vi "Double FFT Mesurament RT with TIME Linearization (Not working mehtod).vi"() -> ()   [LabVIEW 2014]
uses:
  <vilib>/Platform/TimedLoop/XDataNode/timing_clust.ctl
  <vilib>/Platform/TimedLoop/XDataNode/nitl_modes.ctl
  <vilib>/Platform/TimedLoop/XDataNode/wakeup.ctl
  <vilib>/FPGAPlugInAG/sbRIO-9636/niLvFpga_Open_sbRIO-9636.vi
  <vilib>/rvi/interface/common/dynamic/niFpgaDynamicAddResources.vi
  <vilib>/Utility/error.llb/Error Cluster From Error Code.vi
  <vilib>/rvi/errors/niLvFpgaAdjustHostInterfaceError.vi
  <vilib>/rvi/interface/common/niFpgaWaitOnOcc.vi
  <vilib>/FPGAPlugInAG/Dynamic/niLvFpga_Run_Dynamic.vi
  <vilib>/FPGAPlugInAG/Dynamic/niLvFpga_Abort_Dynamic.vi
  <vilib>/FPGAPlugInAG/Dynamic/niLvFpga_Reset_Dynamic.vi
  <vilib>/FPGAPlugInAG/Dynamic/niLvFpga_Close_Dynamic.vi
  <vilib>/rvi/interface/nirviOpenFPGA/nirviOpenFPGA.xnode
  FPGA Bitfiles/LaserDistanceSen_FPGATarget_DoubleFFTMesuram_r82pz3ZO4sk.lvbitx
  FPGA Target/Test VIs/Double FFT Mesurament Test.vi
  <vilib>/rvi/interface/nirviReadWriteControl/nirviReadWriteControl.xnode
  <vilib>/rvi/interface/nirviMethod/nirviMethod.xnode
  <vilib>/Platform/TimedLoop/XDataNode/XDataNode.xnode
  <vilib>/rvi/interface/nirviCloseFPGA/nirviCloseFPGA.xnode
  <vilib>/FPGAPlugInAG/Dynamic/niLvFpga_ConfigureFifo_Dynamic.vi
  <vilib>/rvi/errors/niLvFpgaMergeErrorWithErrorCode.vi
  <vilib>/FPGAPlugInAG/Dynamic/niLvFpga_StartFifo_Dynamic.vi
  <vilib>/rvi/interface/Simulation/niFpgaSimulationCallBeginRW.vi
  <vilib>/FPGAPlugInAG/Dynamic/niLvFpga_ReadFifo_Dynamic.vi
  <vilib>/Platform/TimedLoop/XDataNode/XDNodeRunTimeDep.lvlib
  NiFpgaLv.dll
panel:
  in  "tieni premuto per":i32=1
  out "Not-Extended Period Fal":cluster{"yi":dbl[], "yi":dbl[]}(graph)
  out "Not-Extended Period RIs":cluster{"yi":dbl[], "yi":dbl[]}(graph)
  out "Triangular Signal (ris-fal)":dbl[](graph)
  out "current lin":i32
  out "Triangular Signal (fal-ris)":dbl[](graph)
  out "Period Graph Ris":dbl[][](graph)
  out "Period Graph Fall":dbl[][](graph)
  in  "Acrive Linearization":bool
  out "#Peaks Sig2":i32
  out "#Peaks Sig1":i32
  in  "polynomial order":i32=3
  in  "side points":i32=13
  out "Second Signal SMOOTH":dbl[](graph)
  out "First Signal SMOOTH":dbl[](graph)
  in  "# Measurements for Linearization":i32=10
  in  "stop":bool
  out "maxbin_secondFFT":i32
  out "maxbin_firstFFT":i32
  out "f_rise":dbl
  out "f_fall":dbl
  out "f_mean":dbl
  out "Velocity (m/s)":dbl
  out "Distance (m)":dbl
  in  "Initial Latency points":u32(slide)=10 scale=0.0..1249.0
  out "Second FFT (bin)":dbl[](graph)
  out "Second Signal (points) - Rising Triangular":dbl[](graph)
  out "First FFT (bin)":dbl[](graph)
  out "First Signal (points) - Falling Triangular":dbl[](graph)
  in  "Snapshot":bool
  in  "Windowing":T1(ring)
  in  "first bin":i32=5
  in  "last bin":i32=255
  in  "lower limit 2":u32(slide)=725 scale=625.0..738.0
  in  "lower limit 1":u32(slide)=100 scale=0.0..113.0
  # "WARNING:\nOnce pressed wait untill the end of operation"
  # "OFFLINE parameters"
  # "Max Detection FFT bin range"
  # "S-G Parameter for Smoothing"
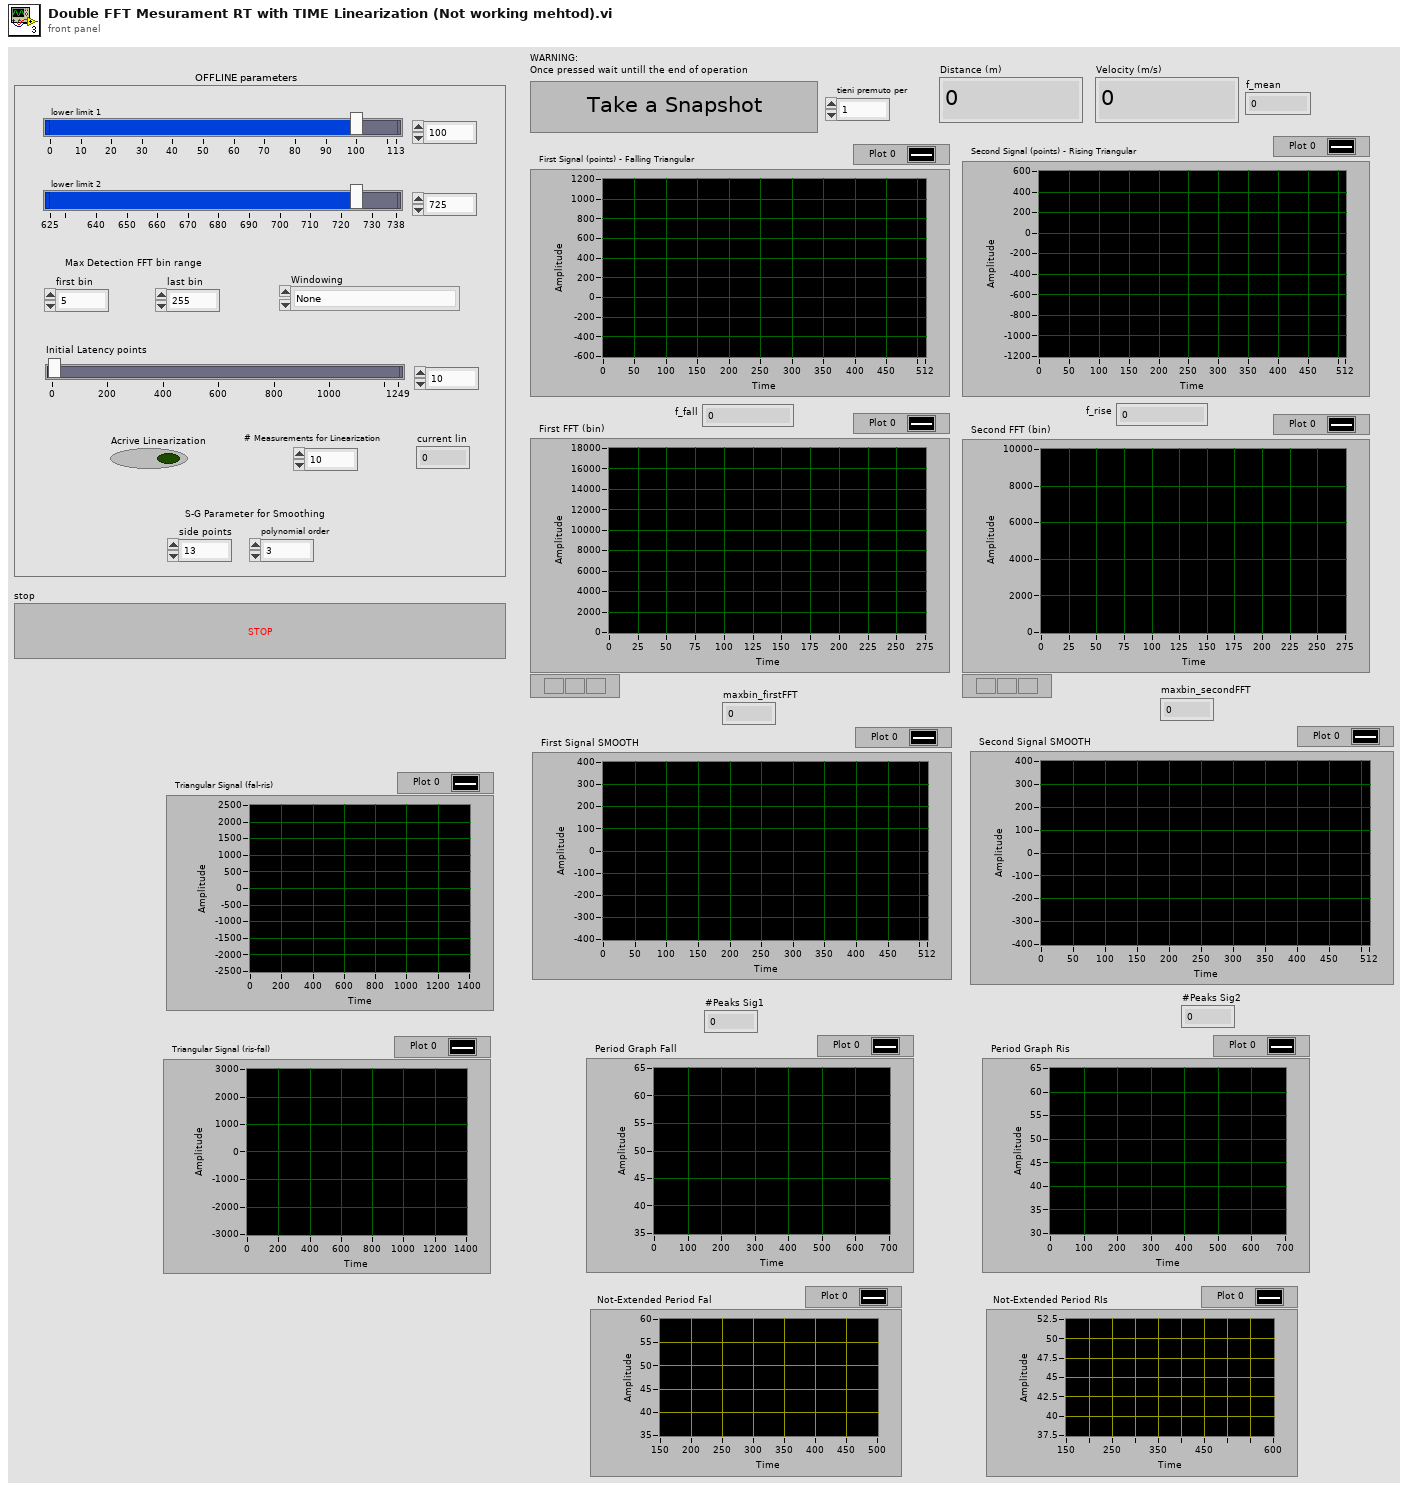
[diagram p1: front panel]
types:
  T1 = enum16{"None", "Hanning", "Hamming", "Blackman", "Blackman-Harris"}
  T2 = typedef "XDNodeRunTimeDep.lvlib/timing_clust.ctl" = cluster{"Expected End [f-1]":u64, "Actual End [f-1]":u64, "Finished Late? [f-1]":bool, "Expected End [i-1]":u64, "Actual End [i-1]":u64, "Finished Late? [i-1]":bool, "Expected Start [i]":u64, "Actual Start [i]":u64, "Expected Start [f]":u64, "Actual Start [f]":u64, "Source Name":string, "Structure Name":string, "Period":i64, "Deadline":i64, "Offset":i64, "Start":i64, "Priority":i32, "Timeout":i32, "Mode":T3, "Wakeup Reason":T4, "Error":errorcluster, "Source Type":string, "Secondary Source Type":string, "Global End Time":u64, "Global Start Time":u64, "Frame Duration":u64, "Iteration Duration":u64, "Assigned CPU":i32, "I/O Scan Engine Mode":u32}
  T3 = typedef "XDNodeRunTimeDep.lvlib/nitl_modes.ctl" = enum32{"No Change", "Process missed periods, maintain original phase", "Discard missed periods, maintain original phase", "Process missed periods, ignore original phase", "Discard missed periods, ignore original phase"}
  T4 = typedef "XDNodeRunTimeDep.lvlib/wakeup.ctl" = enum32{"Normal", "Aborted", "Asynchronous wakeup", "Timing source error", "Timed loop error", "Timeout"}
  T5 = typedef "NI_Matrix.lvlib/RealMatrix.ctl" = dbl[][]
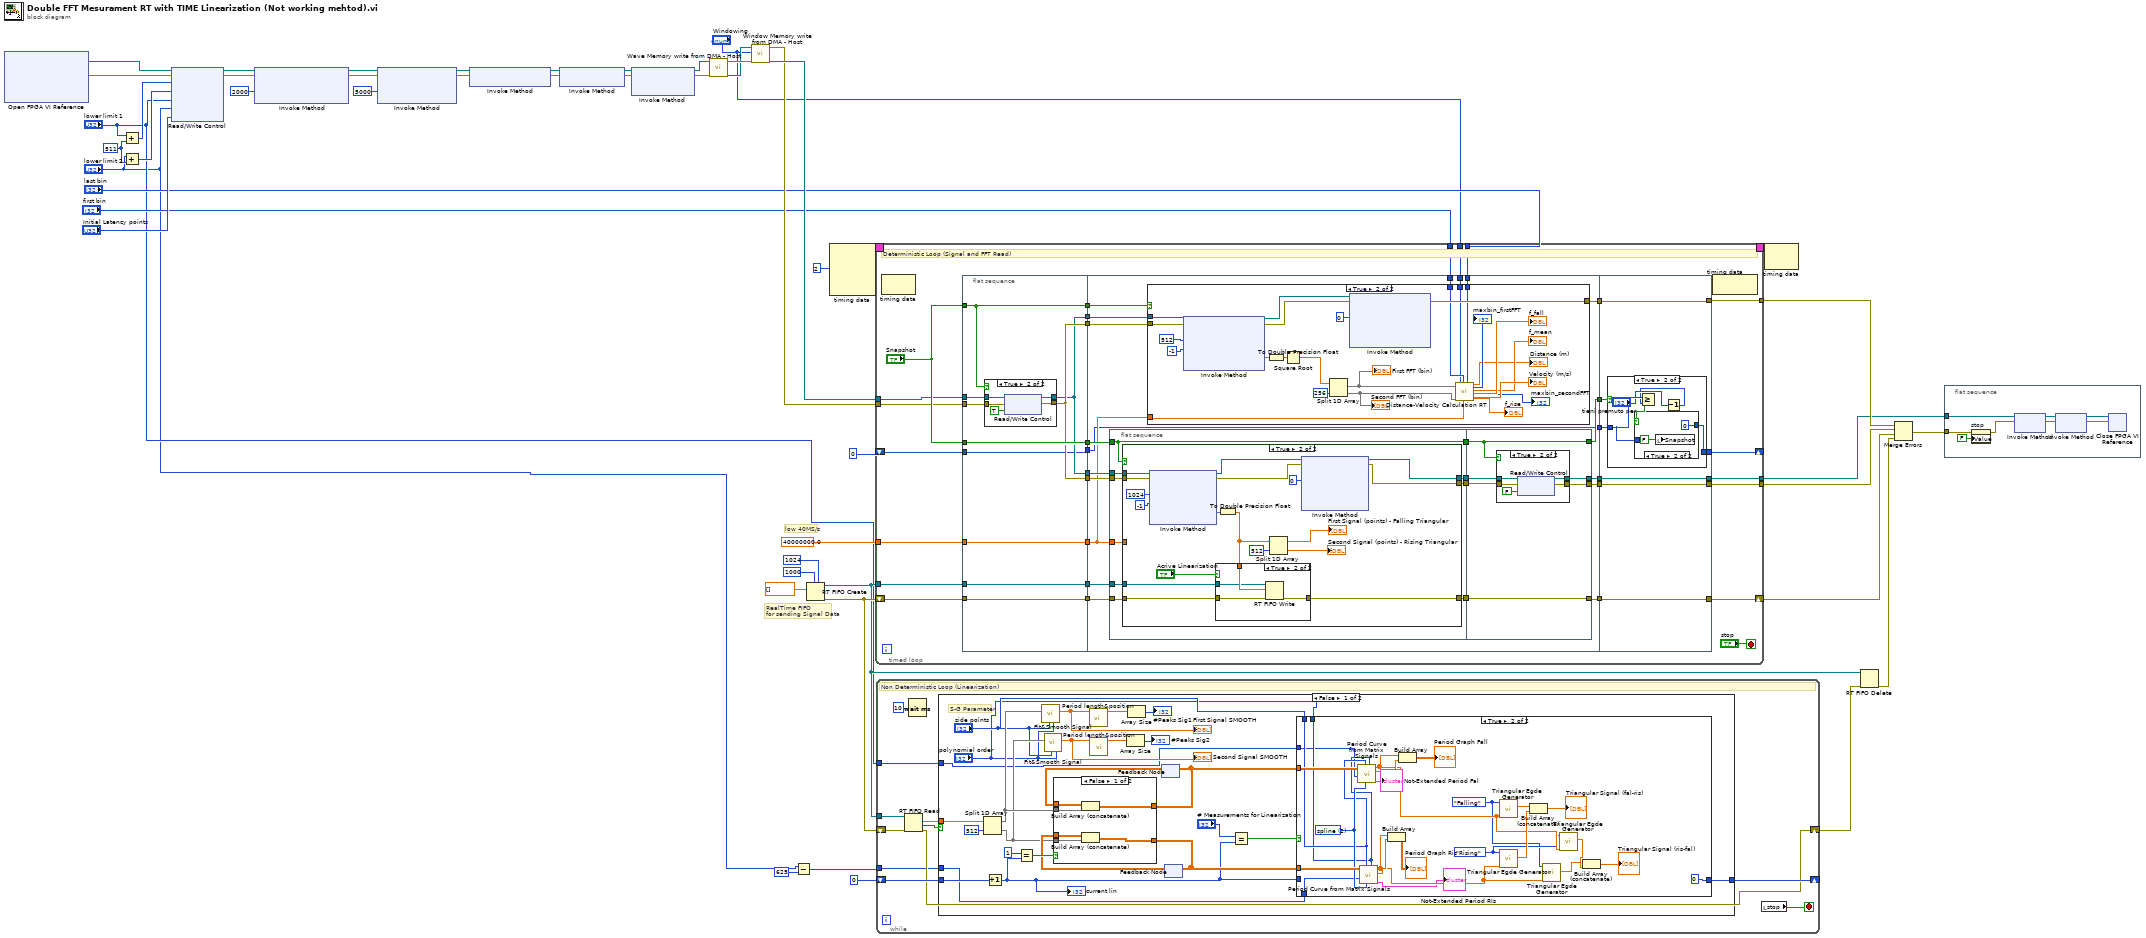
[diagram p0: block diagram]
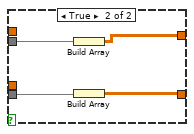
[diagram p3: hidden frame]
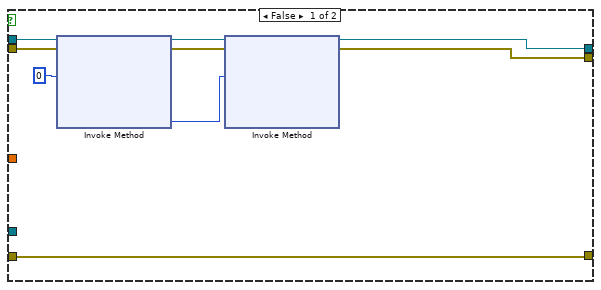
[diagram p6: hidden frame]
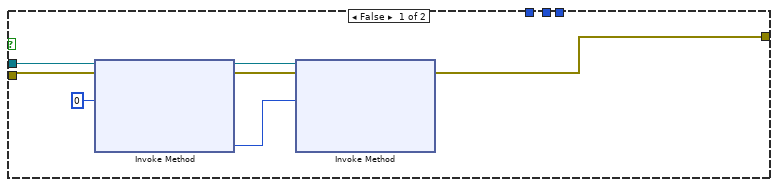
[diagram p9: hidden frame]
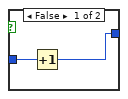
[diagram p11: hidden frame]
diagram:
  w47 = u32 511 ("y")
  # "RealTime FIFO \nfor sending Signal Data"
  # "low 40MS/s"
  n1 = xnode "Open FPGA VI Reference"() -> ("FPGA VI Reference Out"=w46:refnum<k20>, "error out"=w45:errorcluster)  [unwired: 2 in]
  n2 = Add(x="lower limit 1", y=w47) -> (x+y=w49:u32)
  n3 = Add(x="lower limit 2", y=w47) -> (x+y=w48:u32)
  n4 = xnode "Read/Write Control"("FPGA VI Reference In"=w46, "error in"=w45, "upper limit 1"=w49, "upper limit 2"=w48, "lower limit 1"="lower limit 1", "lower limit 2"="lower limit 2", "Latency points"="Initial Latency points") -> ("FPGA VI Reference Out"=w42:refnum<k20>, "error out"=w41:errorcluster)
  n5 = xnode "Invoke Method"("FPGA VI Reference In"=w42, "error in"=w41, "Requested Depth"=u32 2000) -> ("FPGA VI Reference Out"=w20:refnum<k20>, "error out"=w21:errorcluster)  [unwired: 1 out]
  n6 = xnode "Invoke Method"("FPGA VI Reference In"=w20, "error in"=w21, "Requested Depth"=u32 5000) -> ("FPGA VI Reference Out"=w34:refnum<k20>, "error out"=w35:errorcluster)  [unwired: 1 out]
  n7 = xnode "Invoke Method"("FPGA VI Reference In"=w34, "error in"=w35) -> ("FPGA VI Reference Out"=w18:refnum<k20>, "error out"=w19:errorcluster)
  n8 = xnode "Invoke Method"("FPGA VI Reference In"=w18, "error in"=w19) -> ("FPGA VI Reference Out"=w32:refnum<k20>, "error out"=w33:errorcluster)
  n9 = xnode "Invoke Method"("FPGA VI Reference In"=w32, "error in"=w33) -> ("FPGA VI Reference Out"=w38:refnum<k20>, "error out"=w37:errorcluster)  [unwired: 1 in]
  n10 = call "Wave Memory write from DMA - Host.vi"("error in"=w37, "FPGA VI Reference In"=w38) -> ("FPGA VI Reference Out"=w23:refnum<k20>, "error out"=w36:errorcluster)  [unwired: 7 in, 1 out]
  n11 = call "Window Memory write from DMA - Host.vi"("error in"=w36, "Enum"="Windowing", "FPGA VI Reference In"=w23) -> ("FPGA VI Reference Out"=w44:refnum<k20>, "error out"=w43:errorcluster)  [unwired: 5 in, 2 out]
  n12 = Subtract(x="lower limit 2", y=u32 625) -> (x-y=w2:u32)
  n13 = RT FIFO Create(1:dbl[] [] ("double precision float"), 4:u32 1000 ("size (10)"), 6:u32 1024 ("elements in array (1)")) -> (8:w10:refnum<k33>, 11:w12:errorcluster)  [unwired: 5 in, 1 out]
  n14 = node-c288(i64 2 ("Period")) -> (w31:T2)  [unwired: 3 in]
  n15 = timed-loop {
    tunnel: w44 -> [w76]
    tunnel: w43 -> [w77]
    tunnel: [w79] -> w28
    tunnel: 40000000.0 ("Sample Rate (S/s)") -> [w81]
    tunnel: [w80] -> w27
    timing: w31 -> [_]
    timing-out: [_] -> w30
    tunnel: "first bin" -> [w65]
    tunnel: "last bin" -> [w64]
    tunnel: [w62] -> w22
    tunnel: "Windowing" -> [w60]
    shift-right: [w54] -> w13
    shift-left: w12 -> [w56]
    tunnel: w10 -> [w58]
    shift-right: [w50] -> _
    shift-left: 0 -> [w52]
    stop <- "stop" stop-if-true
    # "Deterministic Loop (Signal and FFT Read)"
    n16 = node-c288() -> ()  [unwired: 1 in, 1 out]
    n17 = flat-sequence {
      tunnel: w76 -> [w89]
      tunnel: w77 -> [w90]
      tunnel: "Snapshot" -> [w87]
      tunnel: "Snapshot" -> [w92]
      tunnel: w81 -> [w93]
      tunnel: [w91] -> w75
      tunnel: [w93] -> w74
      tunnel: [w92] -> w73
      tunnel: [w87] -> w72
      tunnel: [w91] -> w71
      tunnel: [w88] -> w70
      tunnel: [w88] -> w69
      tunnel: [w86] -> w59
      tunnel: w58 -> [w86]
      tunnel: [w85] -> w57
      tunnel: w56 -> [w85]
      tunnel: [w84] -> w53
      tunnel: w52 -> [w84]
      tunnel: w75 -> [w118]
      tunnel: w74 -> [w106]
      tunnel: w73 -> [w112]
      tunnel: w72 -> [w115]
      tunnel: w71 -> [w114]
      tunnel: w70 -> [w113]
      tunnel: w69 -> [w119]
      tunnel: [w117] -> w68
      tunnel: [w116] -> w67
      tunnel: [w111] -> w66
      tunnel: w65 -> [w110]
      tunnel: w64 -> [w109]
      tunnel: [w108] -> w61
      tunnel: w60 -> [w107]
      tunnel: w59 -> [w105]
      tunnel: w57 -> [w104]
      tunnel: [w102] -> w55
      tunnel: w53 -> [w101]
      tunnel: [w101] -> w51
      tunnel: [w214] -> w79
      tunnel: [w215] -> w80
      tunnel: w68 -> [w215]
      tunnel: w67 -> [w214]
      tunnel: w66 -> [w213]
      tunnel: [w212] -> w62
      tunnel: w61 -> [w212]
      tunnel: [w211] -> w54
      tunnel: w55 -> [w211]
      tunnel: w51 -> [w210]
      tunnel: [w209] -> w50
      frame #0 {
        n18 = case shown="True" w87 {
          tunnel: [w94 w99] -> w91
          tunnel: w90 -> [w94 w98]
          tunnel: w89 -> [w95 w97]
          tunnel: [w95 w96] -> w88
          frame False {
          }
          frame True {
            n19 = xnode "Read/Write Control"("FPGA VI Reference In"=w97, "error in"=w98, "snapshot"=TRUE) -> ("FPGA VI Reference Out"=w96:refnum<k20>, "error out"=w99:errorcluster)
          }
        }
      }
      frame #1 {
        n20 = flat-sequence {
          tunnel: w119 -> [w131]
          tunnel: w118 -> [w130]
          tunnel: w106 -> [w129]
          tunnel: w112 -> [w126]
          tunnel: [w128] -> w122
          tunnel: [w127] -> w121
          tunnel: [w126] -> w120
          tunnel: w105 -> [w125]
          tunnel: w104 -> [w124]
          tunnel: [w123] -> w103
          tunnel: [w167] -> w116
          tunnel: w122 -> [w169]
          tunnel: w121 -> [w168]
          tunnel: w120 -> [w166]
          tunnel: [w166] -> w111
          tunnel: [w165] -> w108
          tunnel: [w164] -> w102
          tunnel: w103 -> [w164]
          frame #0 {
            n21 = case shown="True" w126 {
              tunnel: w131 -> [w139 w158]
              tunnel: w130 -> [w137 w157]
              tunnel: [w136 w150] -> w127
              tunnel: w129 -> [_ _]
              tunnel: [w133 w149] -> w128
              tunnel: w125 -> [_ w144]
              tunnel: w124 -> [w132 w143]
              tunnel: [w132 w142] -> w123
              frame False {
                n22 = xnode "Invoke Method"("FPGA VI Reference In"=w139, "error in"=w137, "Number of Elements"=u32 0) -> ("FPGA VI Reference Out"=w135:refnum<k20>, "error out"=w134:errorcluster, "Elements Remaining"=w138:u32)  [unwired: 1 in, 1 out]
                n23 = xnode "Invoke Method"("FPGA VI Reference In"=w135, "error in"=w134, "Number of Elements"=w138) -> ("FPGA VI Reference Out"=w133:refnum<k20>, "error out"=w136:errorcluster)  [unwired: 1 in, 2 out]
              }
              frame True {
                n24 = xnode "Invoke Method"("FPGA VI Reference In"=w158, "error in"=w157, "Number of Elements"=u32 1024, "Timeout (ms)"=-1) -> ("FPGA VI Reference Out"=w152:refnum<k20>, "error out"=w151:errorcluster, "Data"=w154:fxp<+/-,12,12>[])  [unwired: 1 out]
                n25 = To Double Precision Float(number=w154) -> (double precision float=w145:dbl[])
                n26 = case shown="True" "Acrive Linearization" {
                  tunnel: w145 -> [_ w163]
                  tunnel: w144 -> [_ w162]
                  tunnel: w143 -> [w159 w161]
                  tunnel: [w159 w160] -> w142
                  frame False {
                  }
                  frame True {
                    n27 = RT FIFO Write(0:w162, 1:w163, 3:w161) -> (11:w160:errorcluster)  [unwired: 2 in, 3 out]
                  }
                }
                n28 = Split 1D Array(array=w145, index=512) -> (first subarray=→"First Signal (points) - Falling Triangular":dbl[], second subarray=→"Second Signal (points) - Rising Triangular":dbl[])
                n29 = xnode "Invoke Method"("FPGA VI Reference In"=w152, "error in"=w151, "Number of Elements"=u32 0) -> ("FPGA VI Reference Out"=w149:refnum<k20>, "error out"=w150:errorcluster)  [unwired: 1 in, 2 out]
              }
            }
          }
          frame #1 {
            n30 = case shown="True" w166 {
              tunnel: [w171 w174] -> w167
              tunnel: w169 -> [w170 w175]
              tunnel: w168 -> [w171 w173]
              tunnel: [w170 w172] -> w165
              frame False {
              }
              frame True {
                n31 = xnode "Read/Write Control"("FPGA VI Reference In"=w175, "error in"=w173, "snapshot"=FALSE) -> ("FPGA VI Reference Out"=w172:refnum<k20>, "error out"=w174:errorcluster)
              }
            }
          }
        }
        n32 = case shown="True" w115 {
          tunnel: w113 -> [w182 w203]
          tunnel: w114 -> [w179 w204]
          tunnel: [w178 w202] -> w117
          tunnel: w110 -> [_ w189]
          tunnel: w109 -> [_ w190]
          tunnel: w107 -> [_ w186]
          tunnel: w106 -> [_ w184]
          frame False {
            n33 = xnode "Invoke Method"("FPGA VI Reference In"=w182, "error in"=w179, "Number of Elements"=u32 0) -> ("FPGA VI Reference Out"=w180:refnum<k20>, "error out"=w177:errorcluster, "Elements Remaining"=w181:u32)  [unwired: 1 in, 1 out]
            n34 = xnode "Invoke Method"("FPGA VI Reference In"=w180, "error in"=w177, "Number of Elements"=w181) -> ("error out"=w178:errorcluster)  [unwired: 1 in, 3 out]
          }
          frame True {
            n35 = xnode "Invoke Method"("FPGA VI Reference In"=w203, "error in"=w204, "Number of Elements"=u32 512, "Timeout (ms)"=-1) -> ("FPGA VI Reference Out"=w200:refnum<k20>, "error out"=w201:errorcluster, "Data"=w206:fxp<+,44,44>[])  [unwired: 1 out]
            n36 = To Double Precision Float(number=w206) -> (double precision float=w205:dbl[])
            n37 = Square Root(x=w205) -> (sqrt(x)=w198:dbl[])
            n38 = Split 1D Array(array=w198, index=256) -> (first subarray=w196:dbl[], second subarray=w195:dbl[])
            "First FFT (bin)" <- w196
            "Second FFT (bin)" <- w195
            n39 = xnode "Invoke Method"("FPGA VI Reference In"=w200, "error in"=w201, "Number of Elements"=u32 0) -> ("error out"=w202:errorcluster)  [unwired: 1 in, 3 out]
            n40 = call "Distance-Velocity Calculation RT.vi"("First FFT"=w196, "Second FFT"=w195, "Windowing"=w186, "first FFT bin"=w189, "Sample Rate (S/s)"=w184, "last FFT bin"=w190) -> ("F_rise"=→"f_rise":dbl, "maxbin_firstFFT"=→"maxbin_firstFFT":i32, "maxbin_secondFFT"=→"maxbin_secondFFT":i32, "Distance (m)"=→"Distance (m)":dbl, "f_mean"=→"f_mean":dbl, "F_fall"=→"f_fall":dbl, "Velocity (m/s)"=→"Velocity (m/s)":dbl)  [unwired: 7 in]
          }
        }
      }
      frame #2 {
        n41 = case shown="True" w213 {
          tunnel: w210 -> [w216 w220]
          tunnel: [w216 w221] -> w209
          frame False {
          }
          frame True {
            n42 = Decrement(x="tieni premuto per") -> (x-1=w217:i32)
            n43 = Greater Or Equal?(x=w220, y=w217) -> (x >= y?=w219:bool)
            n44 = case shown="True" w219 {
              tunnel: w220 -> [w222 _]
              tunnel: [w223 0] -> w221
              frame False {
                n45 = Increment(x=w222) -> (x+1=w223:i32)
              }
              frame True {
                n46 = local write "Snapshot"(FALSE ("Snapshot")) -> ()
              }
            }
          }
        }
      }
    }
    n47 = node-c288() -> ()  [unwired: 1 in, 1 out]
  }
  n48 = while {
    shift-right: [w228] -> w9
    shift-left: w12 -> [w230]
    tunnel: w10 -> [w235]
    shift-right: [w229] -> _
    shift-left: 0 -> [w233]
    tunnel: "lower limit 1" -> [w227]
    tunnel: w2 -> [w226]
    stop <- w234 stop-if-true
    # "Non Deterministic Loop (Linearization)"
    n49 = RT FIFO Read(0:w235, 3:w230) -> (9:w232:dbl[], 10:w231:bool, 11:w228:errorcluster)  [unwired: 2 in, 2 out]
    n50 = Wait (ms)(milliseconds to wait=u32 10 ("millisecond multiple")) -> ()  [unwired: 1 out]
    n51 = case shown="False" w231 {
      tunnel: w233 -> [w261 w297]
      tunnel: [w250 w297] -> w229
      tunnel: w232 -> [w259 _]
      tunnel: w227 -> [w238 _]
      tunnel: w226 -> [w237 _]
      frame False {
        # "S-G Parameter"
        n52 = Split 1D Array(array=w259, index=512) -> (first subarray=w248:dbl[], second subarray=w247:dbl[])
        n53 = Increment(x=w261) -> (x+1=w251:i32)
        "current lin" <- w251
        n54 = Equal?(x=1, y=w251) -> (x = y?=w257:bool)
        n55 = call "Fit&Smooth Signal.vi"("polynomial order"="polynomial order", "side points"="side points", "Signal"=w248) -> ("SmoothFitSignal"=w244:dbl[])  [unwired: 8 in]
        "First Signal SMOOTH" <- w244
        n56 = call "Fit&Smooth Signal.vi"("polynomial order"="polynomial order", "side points"="side points", "Signal"=w247) -> ("SmoothFitSignal"=w243:dbl[])  [unwired: 8 in]
        "Second Signal SMOOTH" <- w243
        n57 = call "Period length&position.vi"("Signal"=w244) -> ("Peak Locations"=w246:dbl[])  [unwired: 9 in, 1 out]
        n58 = call "Period length&position.vi"("Signal"=w243) -> ("Peak Locations"=w245:dbl[])  [unwired: 9 in, 1 out]
        n59 = Array Size(array=w245) -> (size(s)=→"#Peaks Sig2":i32)
        n60 = Array Size(array=w246) -> (size(s)=→"#Peaks Sig1":i32)
        n61 = feedback #1() -> (w256:T5)  [unwired: 1 in]
        n62 = feedback #2() -> (w255:T5)  [unwired: 1 in]
        n63 = case shown="False" w257 {
          tunnel: w247 -> [w291 w294]
          tunnel: w248 -> [w292 w296]
          tunnel: [w290 w293] -> w252
          tunnel: [w289 w295] -> w253
          tunnel: w256 -> [w288 _]
          tunnel: w255 -> [w287 _]
          frame False {
            n64 = Build Array (concatenate)(w288, w292) -> (w289:T5)
            n65 = Build Array (concatenate)(w287, w291) -> (w290:T5)
          }
          frame True {
            n66 = Build Array(w296) -> (w295:T5)
            n67 = Build Array(w294) -> (w293:T5)
          }
        }
        n68 = feedback-in #1(w253) -> ()
        n69 = feedback-in #2(w252) -> ()
        n70 = Equal?(x="# Measurements for Linearization", y=w251) -> (x = y?=w249:bool)
        n71 = case shown="True" w249 {
          tunnel: w253 -> [_ w284]
          tunnel: w252 -> [_ w285]
          tunnel: w251 -> [w262 _]
          tunnel: [w262 0] -> w250
          tunnel: "side points" -> [_ w279]
          tunnel: "polynomial order" -> [_ w278]
          tunnel: w238 -> [_ w265]
          tunnel: w237 -> [_ w264]
          frame False {
          }
          frame True {
            w270 = enum16{"Rising", "Falling"}."Rising" ("Triangular edge")
            w269 = enum16{"Rising", "Falling"}."Falling" ("Triangular edge")
            w283 = 2 items=["nearest", "linear", "spline", "cubic Hermite", "Lagrange"] ("Interpolation Method")
            n72 = call "Period Curve from Matrix Signals.vi"("S-G Polynomial Order"=w278, "Interpolation Method"=w283, "S-G Side Points"=w279, "first_discard_bins"=w265, "Signals Matrix"=w284) -> ("Not-Extended Period Length Curve"=→"Not-Extended Period Fal":cluster{"yi":dbl[], "yi":dbl[]}, "Period Length Curve by  Fitting"=w277:dbl[], "Period Length Curve by Interpolation"=w271:dbl[])  [unwired: 4 in]
            n73 = call "Period Curve from Matrix Signals.vi"("S-G Polynomial Order"=w278, "Interpolation Method"=w283, "S-G Side Points"=w279, "first_discard_bins"=w264, "Signals Matrix"=w285) -> ("Not-Extended Period Length Curve"=→"Not-Extended Period RIs":cluster{"yi":dbl[], "yi":dbl[]}, "Period Length Curve by  Fitting"=w275:dbl[], "Period Length Curve by Interpolation"=w272:dbl[])  [unwired: 4 in]
            n74 = Build Array(w272, w275) -> (→"Period Graph Ris":dbl[][])
            n75 = Build Array(w271, w277) -> (→"Period Graph Fall":dbl[][])
            n76 = call "Triangular Egde Generator.vi"("Sample values"=w271, "Triangular edge"=w269) -> ("Skew Triangular"=w282:dbl[])  [unwired: 9 in]
            n77 = call "Triangular Egde Generator.vi"("Sample values"=w272, "Triangular edge"=w270) -> ("Skew Triangular"=w281:dbl[])  [unwired: 9 in]
            n78 = Build Array (concatenate)(w282, w281) -> (→"Triangular Signal (fal-ris)":dbl[])
            n79 = call "Triangular Egde Generator.vi"("Sample values"=w272, "Triangular edge"=w269) -> ("Skew Triangular"=w267:dbl[])  [unwired: 9 in]
            n80 = call "Triangular Egde Generator.vi"("Sample values"=w271, "Triangular edge"=w270) -> ("Skew Triangular"=w268:dbl[])  [unwired: 9 in]
            n81 = Build Array (concatenate)(w267, w268) -> (→"Triangular Signal (ris-fal)":dbl[])
          }
        }
      }
      frame True {
      }
    }
    n82 = local read "stop"() -> (w234:bool)
  }
  n83 = node-c288(w30) -> ()  [unwired: 1 out]
  n84 = RT FIFO Delete(0:w10, 3:w9) -> (11:w8:errorcluster)  [unwired: 1 in]
  n85 = Merge Errors(w27, w28, w13, w8) -> (w11:errorcluster)
  n86 = flat-sequence {
    tunnel: w11 -> [w301]
    tunnel: w22 -> [w298]
    frame #0 {
      n87 = property on="stop" class="Bool (strict)"(error in=w301, "Value"=FALSE ("stop")) -> (error out=w300:errorcluster)  [unwired: 1 in, 1 out]
      n88 = xnode "Invoke Method"("FPGA VI Reference In"=w298, "error in"=w300) -> ("FPGA VI Reference Out"=w303:refnum<k20>, "error out"=w302:errorcluster)
      n89 = xnode "Invoke Method"("FPGA VI Reference In"=w303, "error in"=w302) -> ("FPGA VI Reference Out"=w304:refnum<k20>, "error out"=w305:errorcluster)
      n90 = xnode "Close FPGA VI Reference"("FPGA VI Reference In"=w304, "error in"=w305) -> ()  [unwired: 1 out]
    }
  }
